vi "Get SMO Name.vi"(8 "error in (no error)":errorcluster, 11 "Inst.FP in":refnum<class "Inst.FP.lvclass">) -> (0 "error out":errorcluster, 2 "SMO Name":string, 3 "Inst.FP out":refnum<class "Inst.FP.lvclass">)   [LabVIEW 2019, in "Inst.FP.lvclass"]
uses:
  Inst.FP.lvclass
  <userlib>/LevyLab/Instrument Framework/Instrument/Instrument.lvclass
  C:/Program Files (x86)/National Instruments/LabVIEW 2019/user.lib/LevyLab/Instrument Framework/Instrument Types/Cryostat/Instrument.Cryostat.lvclass
  C:/Program Files (x86)/National Instruments/LabVIEW 2019/user.lib/LevyLab/Instrument Framework/Instrument/Instrument.lvclass
  C:/Program Files (x86)/National Instruments/LabVIEW 2019/vi.lib/JKI/JKI SMO/SMO/SMO.lvclass
  9c2a333f-09fb-4447-bd3b-ac42ba56788b.vi
  <userlib>/LevyLab/Instrument Framework/Instrument Types/Cryostat/Instrument.Cryostat.lvclass
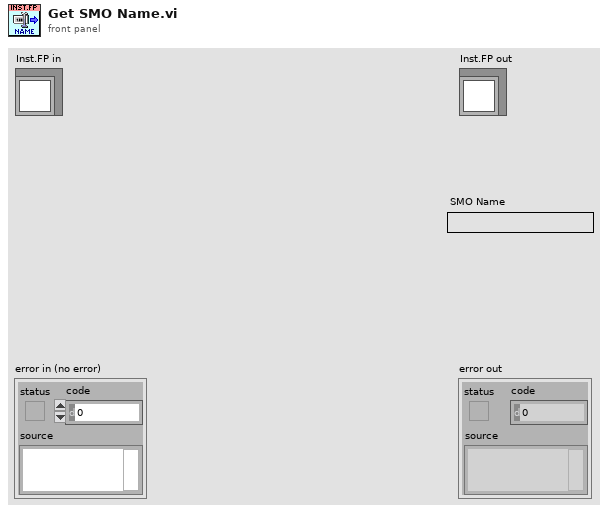
[diagram p1: front panel]
types:
  T1 = typedef "Inst.FP.lvclass/Inst.FP.Type--Enum.ctl" = enum32{"Wet", "CF"}
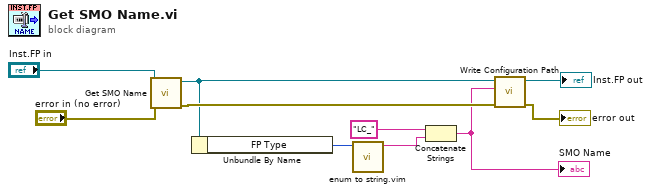
[diagram p0: block diagram]
diagram:
  n1 = call-parent "Get SMO Name.vi"("error in (no error)"="error in (no error)", "Instrument in"="Inst.FP in") -> ("error out"=w7:errorcluster, "Instrument out"=w6:refnum<class "Inst.FP.lvclass">)  [unwired: 7 in, 1 out]
  n2 = Unbundle By Name(w6) -> ("FP Type"=w9:T1)
  n3 = call "enum to string.vim"("enum in"=w9) -> ("string out"=w8:string)  [unwired: 9 in, 1 out]
  n4 = Concatenate Strings("LC_" ("SMO Name"), w8) -> (w2:string)
  "SMO Name" <- w2
  n5 = call <userlib>:"Write Configuration Path.vi"("error in (no error)"=w7, "name or relative path"=w2, "Instrument in"=w6) -> ("error out"=→"error out":errorcluster, "Instrument out"=→"Inst.FP out":refnum<class "Inst.FP.lvclass">)  [unwired: 7 in]
